vi "about.vi"   [LabVIEW 2017]
uses:
  ESLSCDLL.dll
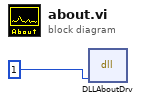
[diagram p0: block diagram]
diagram:
  n1 = dll-call lib="C:/ENTW/PCIE/64bit/lv64/lv64/board.vis/ESLSCDLL.dll" fn="DLLAboutDrv"("drv"=1) -> ()  [unwired: 5 in, 2 out]
